vi "Maximize Window Drop In.vi"(8 "error out 2":errorcluster) -> (0 "error out":errorcluster)   [LabVIEW 2018]
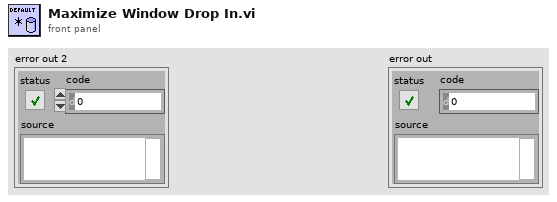
[diagram p1: front panel]
types:
  T1 = enum32{"Invalid", "Standard", "Closed", "Hidden", "Minimized", "Maximized"}
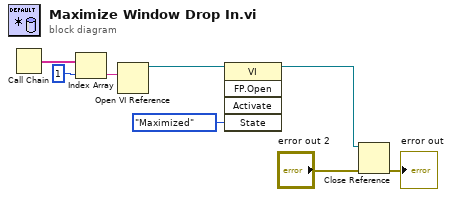
[diagram p0: block diagram]
diagram:
  n1 = Call Chain() -> (call chain=w8:string[])
  n2 = Index Array(array=w8, index=1) -> (element=w6:string)
  n3 = Open VI Reference(vi path=w6) -> (vi reference=w2:refnum<vi>)  [unwired: 5 in, 1 out]
  n4 = invoke class="VI" method="FP.Open"(reference=w2, "State"=T1."Maximized") -> (reference out=w5:refnum<vi>)  [unwired: 3 in, 4 out]
  n5 = Close Reference(reference=w5, error in (no error)="error out 2") -> (error out=→"error out":errorcluster)
